vi "Integration_Test_All_Methods.vi"() -> ()   [LabVIEW 2016]
uses:
  <vilib>/httpClient/LabVIEWHTTPClient.lvlib
  Response/Response.lvclass
panel:
  out "GET":string
  out "GET":dbl
  out "Put":bool
  out "PUT":string="{\n  \"id\": 5,\n  \"name\": \"FIveHUNDRED\",\n  \"age\": \"SIXTYTWO\"\n}"
  out "Patch":bool
  out "Post":bool
  out "Delete":bool
  out "GET":bool
  out "PATCH":string="{\n  \"id\": 5,\n  \"name\": \"Five\",\n  \"age\": \"six\"\n}"
  out "Delete":string="{}"
  out "POST":string="{\n  \"id\": 5,\n  \"name\": \"Five\"\n}"
  out "Get":string="[\n  {\n    \"id\": 0,\n    \"name\": \"Zero\",\n    \"age\": \"Zero\"\n  },\n  {\n    \"id\": 1,\n    \"name\": \"one\",\n    \"age\": \"one\"\n  },\n  {\n    \"id\": 2,\n    \"name\": \"two\",\n    \"age\": \"two\"\n  },\n  {\n    \"id\": 3,\n    \"name\": \"three\",\n    \"age\": \"three\"\n  },\n  {\n    \"id\": 4,\n    \"name\": \"four\",\n    \"age\": \"four\"\n  },\n  {\n    \"id\": 5,\n    \"name\": \"five\"\n  }\n]"
  out "LabVIEW Get":string="[\n  {\n    \"id\": 0,\n    \"name\": \"Zero\",\n    \"age\": \"Zero\"\n  },\n  {\n    \"id\": 1,\n    \"name\": \"one\",\n    \"age\": \"one\"\n  },\n  {\n    \"id\": 2,\n    \"name\": \"two\",\n    \"age\": \"two\"\n  },\n  {\n    \"id\": 3,\n    \"name\": \"three\",\n    \"age\": \"three\"\n  },\n  {\n    \"id\": 4,\n    \"name\": \"four\",\n    \"age\": \"four\"\n  },\n  {\n    \"id\": 5,\n    \"name\": \"FIveHUNDRED\",\n    \"age\": \"SIXTYTWO\"\n  }\n]"
  in  "Path to db.json file":path=path "C:/Users/monke/Desktop/db.json"
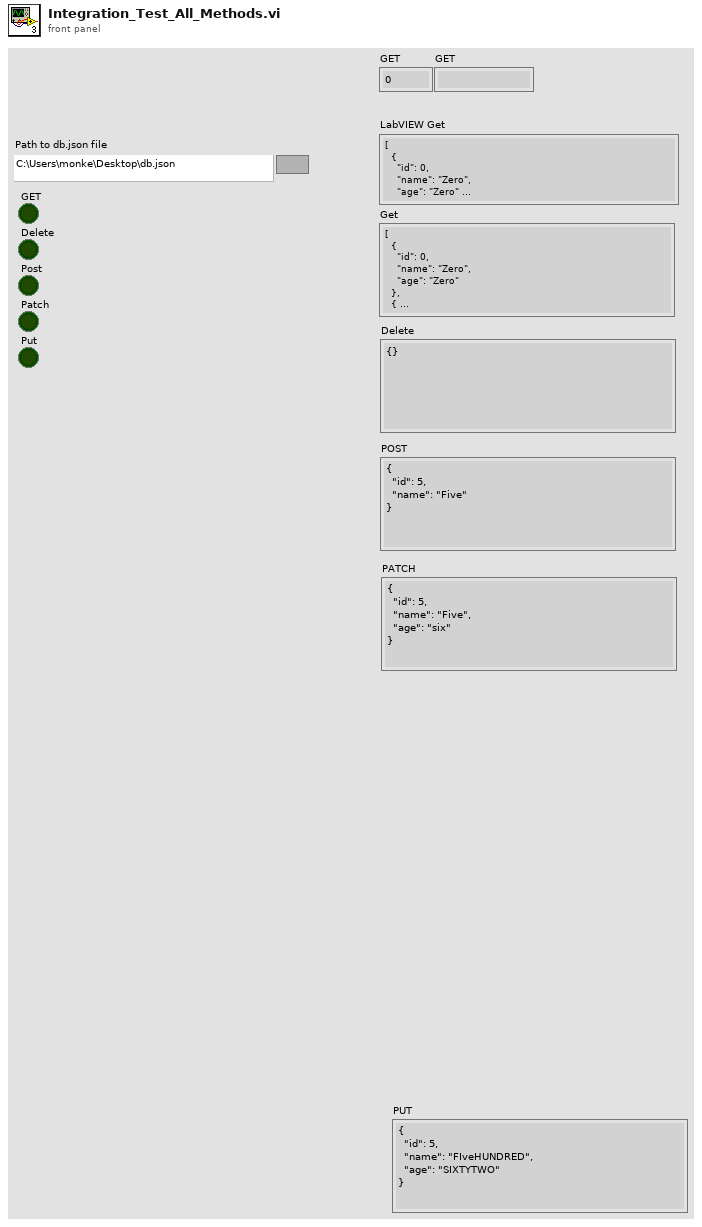
[diagram p1: front panel]
types:
  T1 = enum32{"invalid app kind", "Development System", "Run Time System", "Student Edition", "Embedded LabVIEW", "Evaluation", "Custom"}
  T2 = enum32{"Invalid", "Standard", "Closed", "Hidden", "Minimized", "Maximized"}
  T3 = enum16{"open", "replace", "create", "open or create", "replace or create", "replace or create with confirmation"}
  T4 = cluster{"Core":cluster{"Current VI Reference":refnum<vi>, "Close Panel on Exit?":bool}, "Your Boolean data":bool, "Log":string}
  T5 = cluster{"Current VI Reference":refnum<vi>, "Close Panel on Exit?":bool}
  T6 = typedef "LabVIEWHTTPClient.lvlib/ClientHandle.ctl" = refnum<k1>
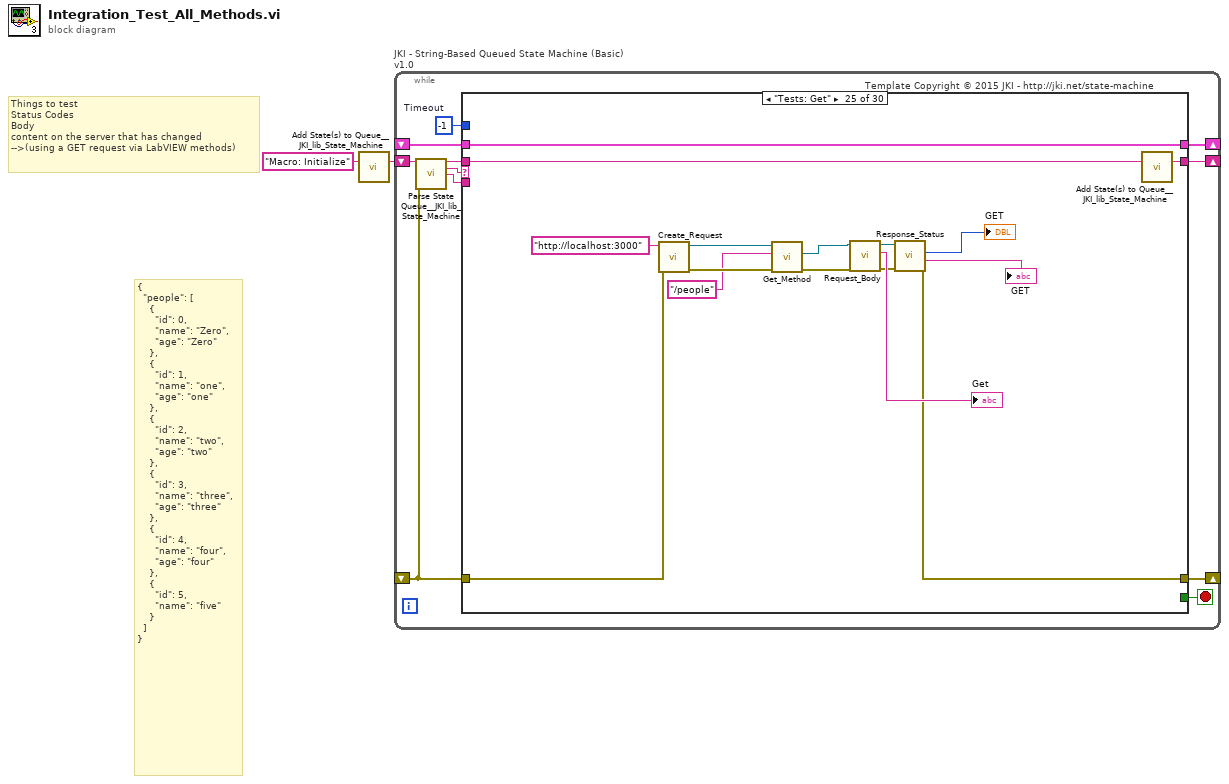
[diagram p0: block diagram]
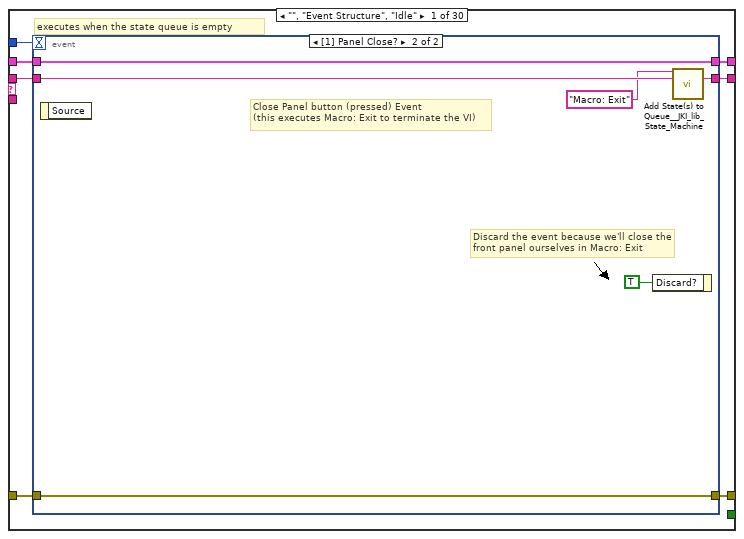
[diagram p2: hidden frame]
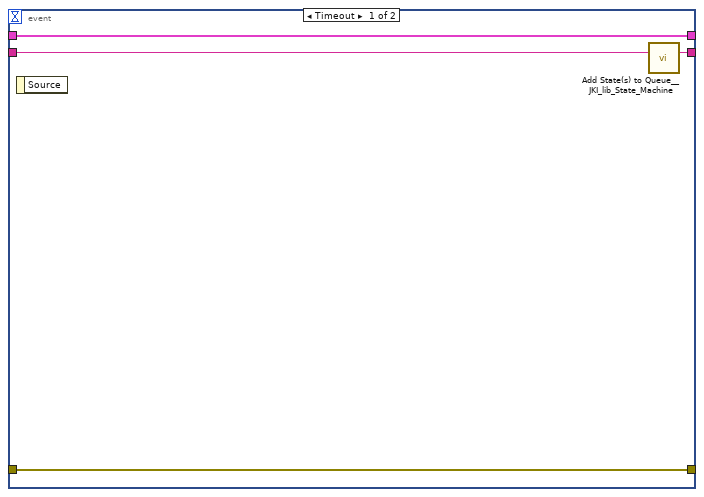
[diagram p3: hidden frame]
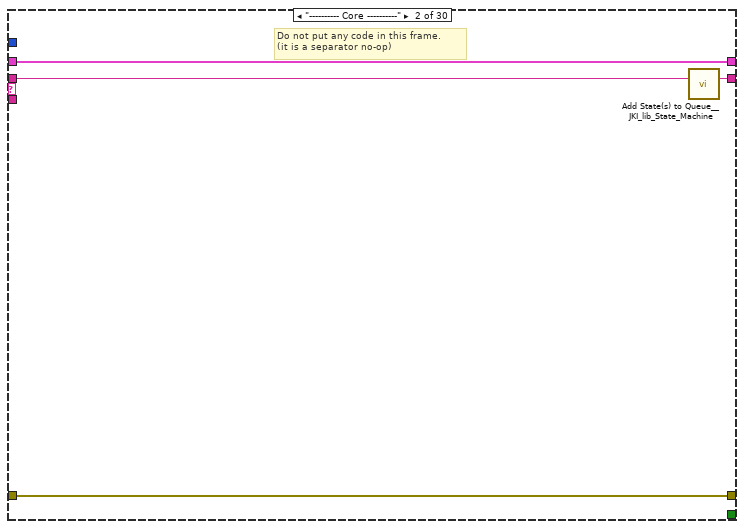
[diagram p4: hidden frame]
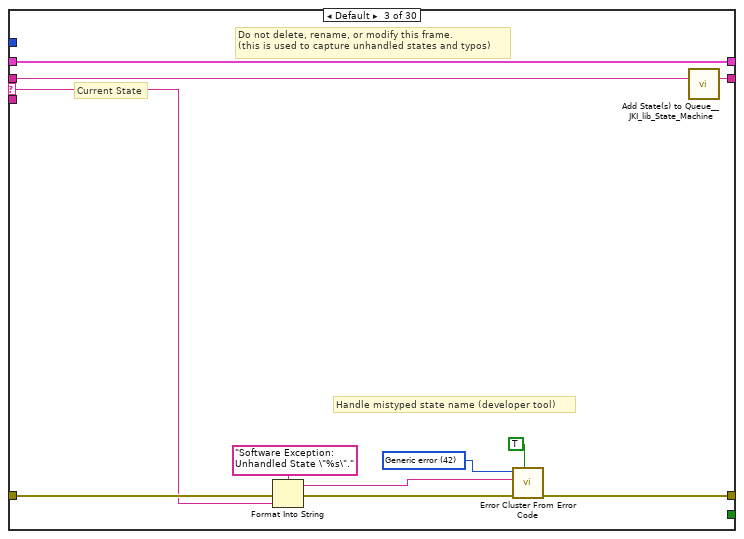
[diagram p5: hidden frame]
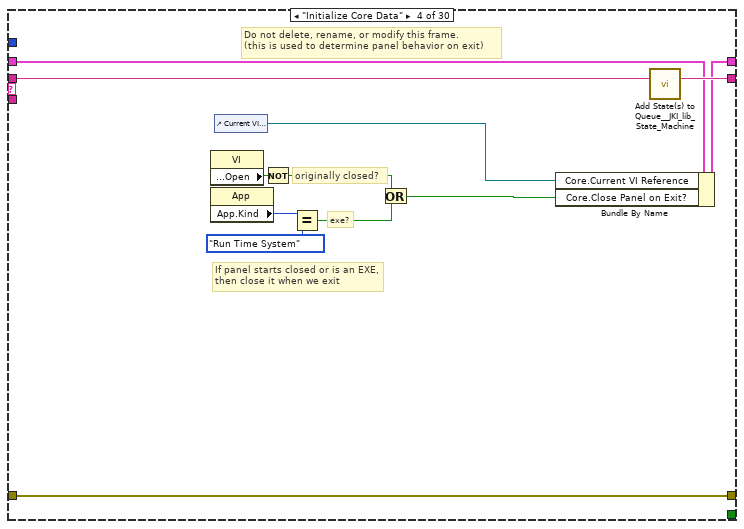
[diagram p6: hidden frame]
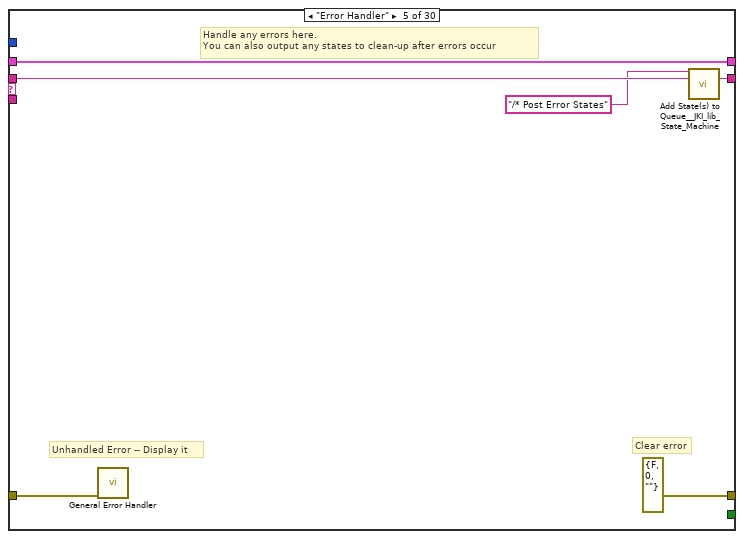
[diagram p7: hidden frame]
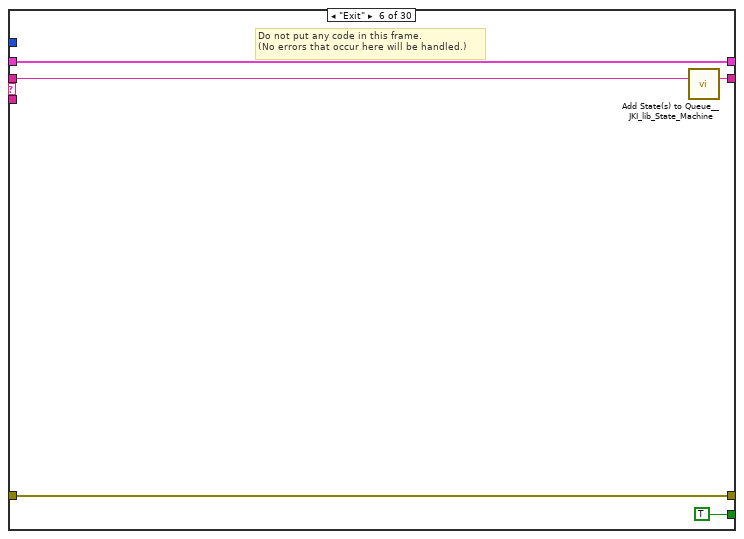
[diagram p8: hidden frame]
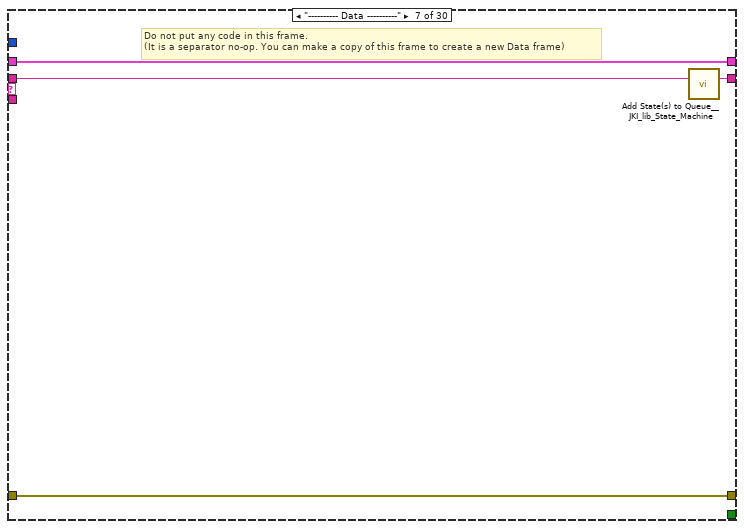
[diagram p9: hidden frame]
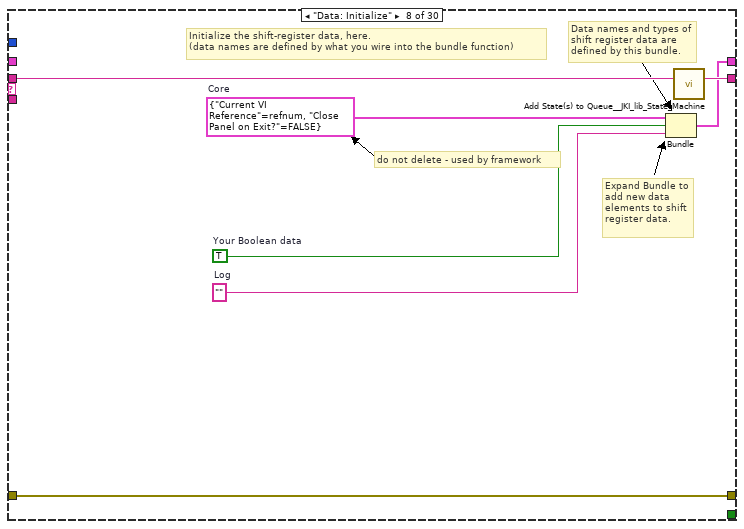
[diagram p10: hidden frame]
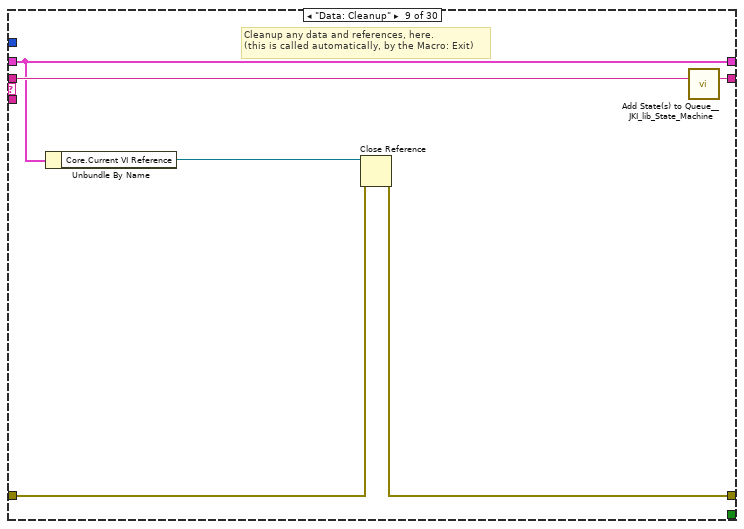
[diagram p11: hidden frame]
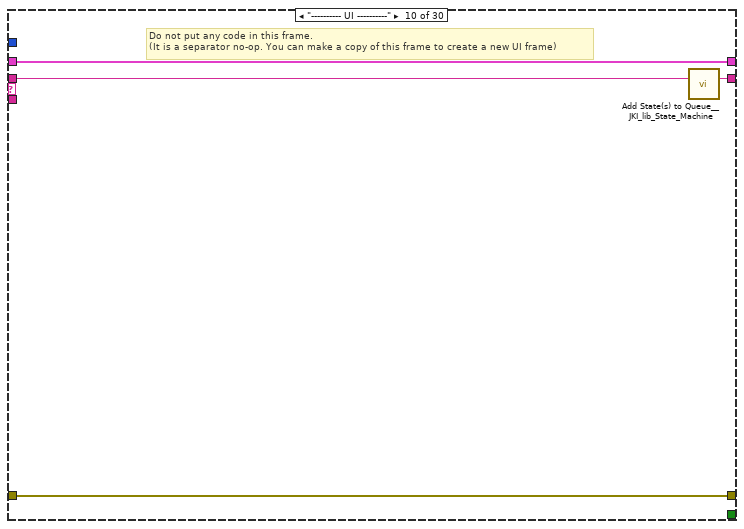
[diagram p12: hidden frame]
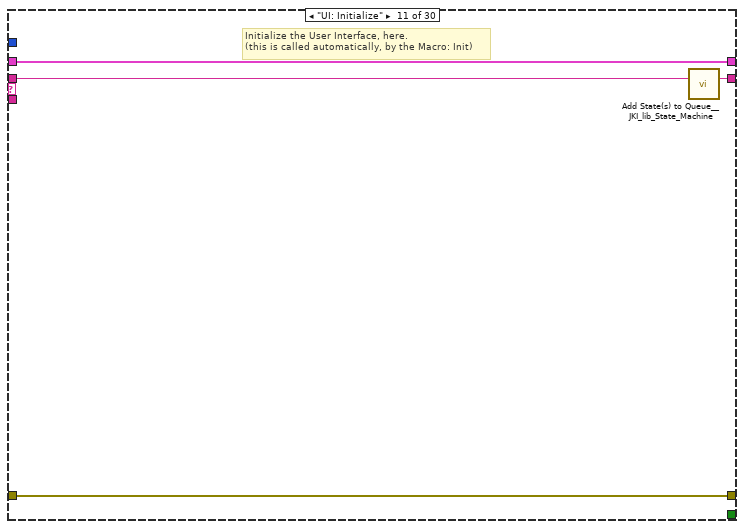
[diagram p13: hidden frame]
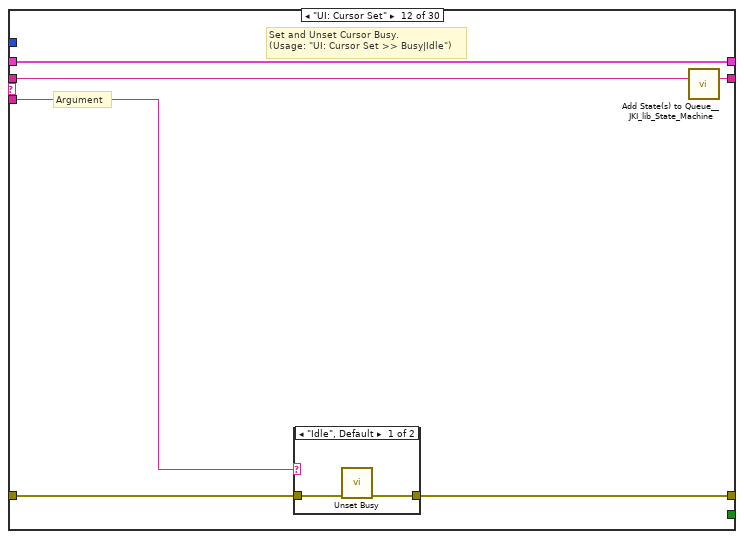
[diagram p14: hidden frame]
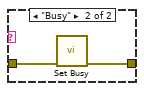
[diagram p15: hidden frame]
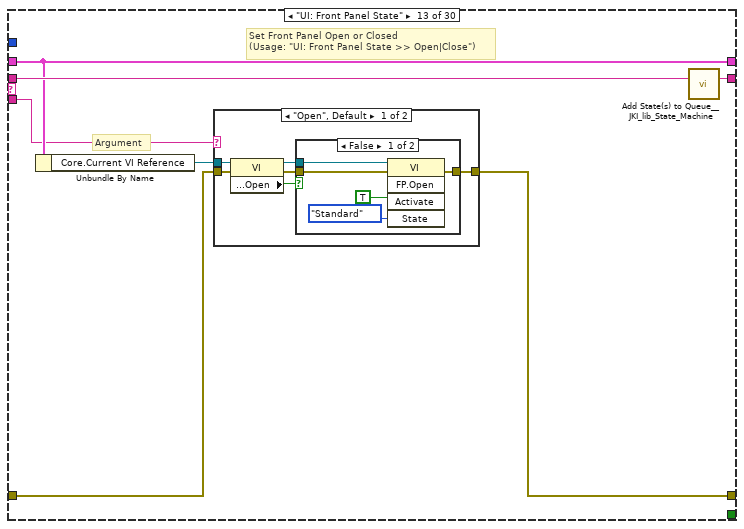
[diagram p16: hidden frame]
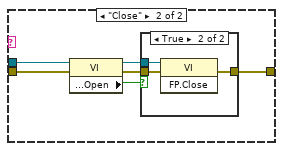
[diagram p18: hidden frame]
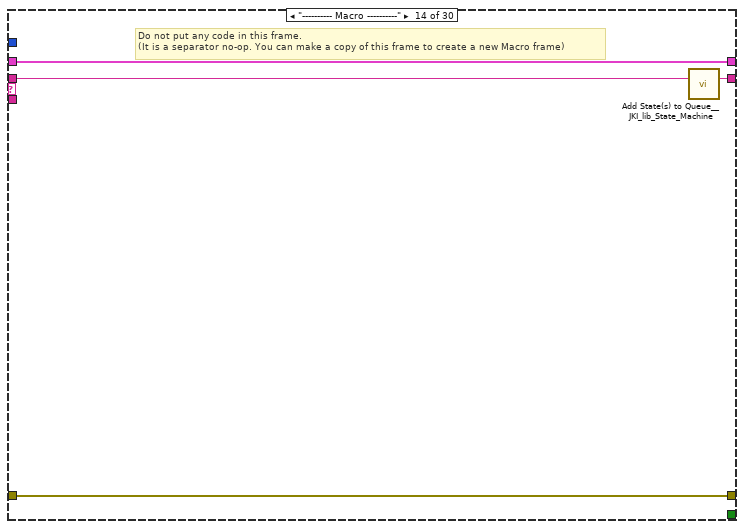
[diagram p20: hidden frame]
diagram:
  # "{\n  \"people\": [\n    {\n      \"id\": 0,\n      \"name\": \"Zero\",\n      \"age\": \"Zero\"\n    },\n    {\n      \"id\": 1,\n      \"name\": \"one\",\n      \"age\": \"one\"\n    },\n    {\n      \"id\": 2,\n      \"name\": \"two\",\n      \"age\": \"two\"\n    },\n    {\n      \"id\": 3,\n      \"name\": \"three\",\n      \"age\": \"three\"\n    },\n    {\n      \"id\": 4,\n      \"name\": \"four\",\n      \"age\": \"four\"\n    },\n    {\n      \"id\": 5,\n      \"name\": \"five\"\n    }\n  ]\n}"
  # "Things to test\nStatus Codes\nBody\ncontent on the server that has changed\n-->(using a GET request via LabVIEW methods)"
  n1 = call <vilib>:"Add State(s) to Queue__JKI_lib_State_Machine.vi"("State(s) in (\"\")"="Macro: Initialize") -> ("States Out"=w2:string)  [unwired: 14 in]
  n2 = while "JKI - String-Based Queued State Machine (Basic) v1.0" {
    shift-right: [w6] -> _
    shift-left: _ -> [w5]
    shift-right: [w9] -> _
    shift-left: _ -> [w3]
    shift-right: [w8] -> _
    shift-left: w2 -> [w10]
    stop <- w7 stop-if-true
    w4 = -1  # Timeout
    # "Template Copyright © 2015 JKI - http://jki.net/state-machine"
    n3 = call <vilib>:"Parse State Queue__JKI_lib_State_Machine.vi"("State Queue"=w10, "Error In (no error)"=w3) -> ("Remaining States"=w12:string, "Current State"=w13:string, "Arguments"=w11:string)  [unwired: 11 in]
    n4 = case shown="\"Tests: Get\"" w13 {
      selector: w13 -> [_ _ w35 _ _ _ _ _ _ _ _ _ _ _ _ _ _ _ _ _ _ _ _ _ _ _ _ _ _ _]
      tunnel: w12 -> [w20 w34 w39 w57 w63 w68 w72 w79 w85 w89 w93 w99 w110 w136 w141 w146 w156 w160 w172 w183 w187 w191 w203 w222 w238 w250 w264 w278 w292 w296]
      tunnel: w11 -> [_ _ _ _ _ _ _ _ _ _ _ w94 w104 _ _ _ _ _ _ _ _ _ w194 _ _ _ _ _ _ _]
      tunnel: w5 -> [w18 w31 w37 w48 w60 w66 w69 _ w80 w86 w91 w97 w106 w133 w138 w143 w153 w158 w170 w181 w184 w188 w192 w219 w225 w248 w262 w276 w290 w293]
      tunnel: [w17 w32 w41 w54 errorcluster {"status"=FALSE, "code"=0, "source"=""} ("error out") w65 w70 w76 w81 w87 w90 w95 w107 w134 w139 w144 w154 w157 w161 w173 w185 w189 w196 w220 w226 w239 w253 w265 w279 w294] -> w9
      tunnel: w3 -> [w16 w32 w40 w54 w59 w65 w70 w76 w82 w87 w90 w96 w108 w134 w139 w144 w154 w157 w162 w174 w185 w189 w197 w220 w233 w240 w254 w266 w280 w294]
      tunnel: [w19 w33 w38 w56 w62 w67 w71 w78 w84 w88 w92 w98 w109 w135 w140 w145 w155 w159 w171 w182 w186 w190 w202 w221 w237 w249 w263 w277 w291 w295] -> w8
      tunnel: [_ _ _ _ _ TRUE _ _ _ _ _ _ _ _ _ _ _ _ _ _ _ _ _ _ _ _ _ _ _ _] -> w7
      tunnel: [w15 w31 w37 w55 w60 w66 w69 w77 w80 w86 w91 w97 w106 w133 w138 w143 w153 w158 w170 w181 w184 w188 w192 w219 w225 w248 w262 w276 w290 w293] -> w6
      tunnel: w4 -> [w14 _ _ _ _ _ _ _ _ _ _ _ _ _ _ _ _ _ _ _ _ _ _ _ _ _ _ _ _ _]
      frame "", "Event Structure", "Idle" {
        # "executes when the state queue is empty"
        n5 = event shown="[1] Panel Close?" {
          selector: _ -> [_ _]
          dyn-events: _ -> [_ _]
          timeout: w14 -> [_ _]
          tunnel: w20 -> [w24 w30]
          tunnel: [w23 w29] -> w19
          tunnel: w18 -> [w21 w27]
          tunnel: [w22 w28] -> w17
          tunnel: w16 -> [w22 w28]
          tunnel: [w21 w27] -> w15
          event Timeout {
            n6 = event-data() -> ()  [unwired: 1 in, 1 out]
            n7 = call <vilib>:"Add State(s) to Queue__JKI_lib_State_Machine.vi"("State(s) in (\"\")"=w24) -> ("States Out"=w23:string)  [unwired: 14 in]
          }
          event Panel Close? {
            # "Discard the event because we'll close the front panel ourselves in Macro: Exit"
            # "Close Panel button (pressed) Event\n(this executes Macro: Exit to terminate the VI)"
            n8 = event-data() -> ()  [unwired: 1 in, 1 out]
            n9 = event-data("Discard?"=TRUE) -> ()  [unwired: 1 in, 1 out]
            n10 = call <vilib>:"Add State(s) to Queue__JKI_lib_State_Machine.vi"("State(s) in Front (\"\")"="Macro: Exit", "State(s) in (\"\")"=w30) -> ("States Out"=w29:string)  [unwired: 13 in]
          }
        }
      }
      frame "---------- Core ----------" {
        # "Do not put any code in this frame.\n(it is a separator no-op)"
        n11 = call <vilib>:"Add State(s) to Queue__JKI_lib_State_Machine.vi"("State(s) in (\"\")"=w34) -> ("States Out"=w33:string)  [unwired: 14 in]
      }
      frame Default {
        w44 = 42 items=["No error", "Argument error", "Memory is full", "Out of zone", "End of file", "File already open", "Generic file I/O error", "File not found", "File permission error", "Disk is full", "Duplicate path", "Too many files open", "System feature not enabled", "Resource file not found", "Cannot add resource", "Resource not found", "Image not found", "Image memory error", "Pen does not exist", "Config type invalid", "Config token not found", "Config parse error", "Config memory error", "Bad external code format", "Bad external code offset", "External code not present", "Null window", "Destroy window error", "Null menu", "Print aborted", "Bad print record", "Print driver error", "Windows error during printing", "Memory error during printing", "Print dialog error", "Generic print error", "Invalid device refnum", "Device not found", "Device parameter error", "Device unit error", "Cannot open device", "Device call aborted", "Generic error", "Cancelled by user", "Object ID too low", "Object ID too high", "Object not in heap", "Unknown heap", "Unknown object (invalid DefProc)", "Unknown object (DefProc not in table)", "Message out of range", "Invalid (null) method", "Unknown message", "Manager call not supported", "Bad address", "Network operation in progress", "Network operation timed out", "Connection is busy", "Network attribute not supported", "Network error", "Address in use", "System out of memory", "Connection aborted", "Connection refused", "Not connected", "Already connected", "Connection closed", "Initialization error (interapplication manager)", "Bad occurrence", "Wait on unbound occurrence handler", "Occurrence queue overflow", "Datalog type conflict", "Unused", "Unrecognized type (interapplication manager)", "Memory corrupt", "Failed to make temporary DLL", "Old CIN version", "Drag socket not found", "Failed to load drop-object", "Failed to register OLE object", "Failed to release OLE object", "Format specifier type mismatch", "Unknown format specifier", "Too few format specifiers", "Too many format specifiers", "Scan failed", "Newer CIN version", "Error converting to variant", "Runtime menu error", "Password tampered", "Variant attribute not found", "Incompatible variant data type", "Event data is not available", "Event Store is not present", "Occurrence is not found", "Event Queue is not created", "Event info is not available", "Refnum passed is NULL", "Error retrieving Class GUID", "Error retrieving CoClass GUID", "Error retrieving TypeLib GUID.", "Bad built application magic bytes.", "Specific driver is different from the specific driver associated with the Logical Name.", "There is no session opened to the class driver.", "Max Error", "MAX - Error with config objects", "MAX - Error loading configuration", "MAX - Group not supported"]
        # "Current State"
        # "Do not delete, rename, or modify this frame.\n(this is used to capture unhandled states and typos)"
        # "Handle mistyped state name (developer tool)"
        n12 = Format Into String(format string="Software Exception: Unhandled State \"%s\"." ("message"), error in=w40, w35) -> (resulting string=w43:string, error out=w42:errorcluster)  [unwired: 1 in]
        n13 = call <vilib>:"Error Cluster From Error Code.vi"("show call chain? (False)"=TRUE, "error in (no error)"=w42, "error message (\"\")"=w43, "error code (0)"=w44) -> ("error out"=w41:errorcluster)  [unwired: 5 in]
        n14 = call <vilib>:"Add State(s) to Queue__JKI_lib_State_Machine.vi"("State(s) in (\"\")"=w39) -> ("States Out"=w38:string)  [unwired: 14 in]
      }
      frame "Initialize Core Data" {
        # "Do not delete, rename, or modify this frame.\n(this is used to determine panel behavior on exit)"
        # "originally closed?"
        # "exe?"
        # "If panel starts closed or is an EXE, then close it when we exit"
        n15 = property class="VI"() -> ("Front Panel.Open"=w53:bool)  [unwired: 2 in, 2 out]
        n16 = property class="App"() -> ("App.Kind"=w52:T1)  [unwired: 2 in, 2 out]
        n17 = control-ref of="Current VI Reference"() -> (w46:refnum<vi>)
        n18 = Not(x=w53) -> (.not. x?=w50:bool)
        n19 = Equal?(x=w52, y=T1."Run Time System" ("Application:Kind")) -> (x = y?=w49:bool)
        n20 = Or(x=w50, y=w49) -> (x .or. y?=w47:bool)
        n21 = Bundle By Name(cluster=w48, "Core.Current VI Reference"=w46, "Core.Close Panel on Exit?"=w47) -> (w55:T4)
        n22 = call <vilib>:"Add State(s) to Queue__JKI_lib_State_Machine.vi"("State(s) in (\"\")"=w57) -> ("States Out"=w56:string)  [unwired: 14 in]
      }
      frame "Error Handler" {
        # "Unhandled Error -- Display it"
        # "Handle any errors here.\nYou can also output any states to clean-up after errors occur"
        # "Clear error"
        n23 = call <vilib>:"General Error Handler.vi"("error in (no error)"=w59) -> ()  [unwired: 10 in, 5 out]
        n24 = call <vilib>:"Add State(s) to Queue__JKI_lib_State_Machine.vi"("State(s) in Front (\"\")"="/* Post Error States", "State(s) in (\"\")"=w63) -> ("States Out"=w62:string)  [unwired: 13 in]
      }
      frame "Exit" {
        # "Do not put any code in this frame.\n(No errors that occur here will be handled.)"
        n25 = call <vilib>:"Add State(s) to Queue__JKI_lib_State_Machine.vi"("State(s) in (\"\")"=w68) -> ("States Out"=w67:string)  [unwired: 14 in]
      }
      frame "---------- Data ----------" {
        # "Do not put any code in this frame.\n(It is a separator no-op. You can make a copy of this frame to create a new Data frame)"
        n26 = call <vilib>:"Add State(s) to Queue__JKI_lib_State_Machine.vi"("State(s) in (\"\")"=w72) -> ("States Out"=w71:string)  [unwired: 14 in]
      }
      frame "Data: Initialize" {
        w73 = T5 {"Current VI Reference"=refnum, "Close Panel on Exit?"=FALSE}  # Core
        w75 = TRUE  # Your Boolean data
        w74 = ""  # Log
        # "do not delete - used by framework"
        # "Expand Bundle to add new data elements to shift register data."
        # "Data names and types of shift register data are defined by this bundle."
        # "Initialize the shift-register data, here.\n(data names are defined by what you wire into the bundle function)"
        n27 = Bundle("Core"=w73, "Your Boolean data"=w75, "Log"=w74) -> (w77:T4)  [unwired: 1 in]
        n28 = call <vilib>:"Add State(s) to Queue__JKI_lib_State_Machine.vi"("State(s) in (\"\")"=w79) -> ("States Out"=w78:string)  [unwired: 14 in]
      }
      frame "Data: Cleanup" {
        # "Cleanup any data and references, here.\n(this is called automatically, by the Macro: Exit)"
        n29 = Unbundle By Name(w80) -> ("Core.Current VI Reference"=w83:refnum<vi>)
        n30 = Close Reference(reference=w83, error in (no error)=w82) -> (error out=w81:errorcluster)
        n31 = call <vilib>:"Add State(s) to Queue__JKI_lib_State_Machine.vi"("State(s) in (\"\")"=w85) -> ("States Out"=w84:string)  [unwired: 14 in]
      }
      frame "---------- UI ----------" {
        # "Do not put any code in this frame.\n(It is a separator no-op. You can make a copy of this frame to create a new UI frame)"
        n32 = call <vilib>:"Add State(s) to Queue__JKI_lib_State_Machine.vi"("State(s) in (\"\")"=w89) -> ("States Out"=w88:string)  [unwired: 14 in]
      }
      frame "UI: Initialize" {
        # "Initialize the User Interface, here.\n(this is called automatically, by the Macro: Init)"
        n33 = call <vilib>:"Add State(s) to Queue__JKI_lib_State_Machine.vi"("State(s) in (\"\")"=w93) -> ("States Out"=w92:string)  [unwired: 14 in]
      }
      frame "UI: Cursor Set" {
        # "Argument"
        # "Set and Unset Cursor Busy.\n(Usage: \"UI: Cursor Set >> Busy|Idle\")"
        n34 = case shown="\"Idle\", Default" w94 {
          tunnel: w96 -> [w101 w103]
          tunnel: [w100 w102] -> w95
          frame "Idle", Default {
            n35 = call <vilib>:"Unset Busy.vi"("error in (no error)"=w101) -> ("error out"=w100:errorcluster)  [unwired: 10 in]
          }
          frame "Busy" {
            n36 = call <vilib>:"Set Busy.vi"("error in (no error)"=w103) -> ("error out"=w102:errorcluster)  [unwired: 9 in, 1 out]
          }
        }
        n37 = call <vilib>:"Add State(s) to Queue__JKI_lib_State_Machine.vi"("State(s) in (\"\")"=w99) -> ("States Out"=w98:string)  [unwired: 14 in]
      }
      frame "UI: Front Panel State" {
        # "Argument"
        # "Set Front Panel Open or Closed\n(Usage: \"UI: Front Panel State >> Open|Close\")"
        n38 = Unbundle By Name(w106) -> ("Core.Current VI Reference"=w105:refnum<vi>)
        n39 = case shown="\"Open\", Default" w104 {
          tunnel: w108 -> [w114 w127]
          tunnel: [w116 w128] -> w107
          tunnel: w105 -> [w115 w125]
          frame "Open", Default {
            n40 = property class="VI"(reference=w115, error in=w114) -> (reference out=w112:refnum<vi>, error out=w113:errorcluster, "Front Panel.Open"=w111:bool)
            n41 = case shown="False" w111 {
              tunnel: [w119 w122] -> w116
              tunnel: w113 -> [w118 w122]
              tunnel: w112 -> [w117 _]
              frame False {
                n42 = invoke class="VI" method="FP.Open"(reference=w117, error in=w118, "Activate"=TRUE, "State"=T2."Standard") -> (error out=w119:errorcluster)  [unwired: 1 in, 4 out]
              }
              frame True {
              }
            }
          }
          frame "Close" {
            n43 = property class="VI"(reference=w125, error in=w127) -> (reference out=w124:refnum<vi>, error out=w126:errorcluster, "Front Panel.Open"=w123:bool)
            n44 = case shown="True" w123 {
              tunnel: [w129 w132] -> w128
              tunnel: w126 -> [w129 w131]
              tunnel: w124 -> [_ w130]
              frame False {
              }
              frame True {
                n45 = invoke class="VI" method="FP.Close"(reference=w130, error in=w131) -> (error out=w132:errorcluster)  [unwired: 1 in, 2 out]
              }
            }
          }
        }
        n46 = call <vilib>:"Add State(s) to Queue__JKI_lib_State_Machine.vi"("State(s) in (\"\")"=w110) -> ("States Out"=w109:string)  [unwired: 14 in]
      }
      frame "---------- Macro ----------" {
        # "Do not put any code in this frame.\n(It is a separator no-op. You can make a copy of this frame to create a new Macro frame)"
        n47 = call <vilib>:"Add State(s) to Queue__JKI_lib_State_Machine.vi"("State(s) in (\"\")"=w136) -> ("States Out"=w135:string)  [unwired: 14 in]
      }
      frame "Macro: Initialize" {
        w137 = "Data: Initialize\nInitialize Core Data\nUI: Initialize\nJsonServer: Create_File\nJsonServer: Run\nUI: Front Panel State >> Open\nMacro: Run Tests"  # Data: Initialize Initialize Core Data UI: Initialize JsonServer: Create_File JsonServer: Run UI: Front Panel State >> Open Macro: Run Tests
        # "Initialization Macro\n(This is called once, when the VI starts)"
        n48 = call <vilib>:"Add State(s) to Queue__JKI_lib_State_Machine.vi"("State(s) in Front (\"\")"=w137, "State(s) in (\"\")"=w141) -> ("States Out"=w140:string)  [unwired: 13 in]
      }
      frame "Macro: Run Tests" {
        # "Do not put any code in this frame.\n(It is a separator no-op. You can make a copy of this frame to create a new Macro frame)"
        n49 = call <vilib>:"Add State(s) to Queue__JKI_lib_State_Machine.vi"("State(s) in Front (\"\")"="Tests: Get\nLabVIEW: Get>>get\nTests: Delete\nLabVIEW: Get>>delete\nTests: Post\nLabVIEW: Get>>post\nTests: Patch\nLabVIEW: Get>>patch\nTests: Put\nLabVIEW: Get>>put\n//Tests: Head", "State(s) in (\"\")"=w146) -> ("States Out"=w145:string)  [unwired: 13 in]
      }
      frame "Macro: Exit" {
        # "Exit Macro\n(This is called once, when the VI exits)"
        n50 = Unbundle By Name(w153) -> ("Core.Close Panel on Exit?"=w152:bool)
        n51 = Select(t="UI: Front Panel State >> Close", s=w152, f="") -> (s? t:f=w149:string)
        n52 = call <vilib>:"Add State(s) to Queue__JKI_lib_State_Machine.vi"("State(s) in (\"\")"=w149, "State(s) at Back (\"\")"="Data: Cleanup\nExit") -> ("States Out"=w147:string)  [unwired: 13 in]
        n53 = call <vilib>:"Add State(s) to Queue__JKI_lib_State_Machine.vi"("State(s) in Front (\"\")"=w147, "State(s) in (\"\")"=w156) -> ("States Out"=w155:string)  [unwired: 13 in]
      }
      frame "---------- JsonServer ----------" {
        n54 = call <vilib>:"Add State(s) to Queue__JKI_lib_State_Machine.vi"("State(s) in (\"\")"=w160) -> ("States Out"=w159:string)  [unwired: 14 in]
      }
      frame "JsonServer: Create_File" {
        n55 = Open/Create/Replace File(file path (use dialog)=path "C:/Users/monke/Desktop/db.json", error in=w162, operation (0:open)=T3."replace or create") -> (refnum out=w166:refnum<file>, error out=w163:errorcluster)  [unwired: 3 in, 1 out]
        n56 = Write to Text File(file (use dialog)=w166, text="{\n  \"people\": [\n    {\n      \"id\": 0,\n      \"name\": \"Zero\",\n      \"age\": \"Zero\"\n    },\n    {\n      \"id\": 1,\n      \"name\": \"one\",\n      \"age\": \"one\"\n    },\n    {\n      \"id\": 2,\n      \"name\": \"two\",\n      \"age\": \"two\"\n    },\n    {\n      \"id\": 3,\n      \"name\": \"three\",\n      \"age\": \"three\"\n    },\n    {\n      \"id\": 4,\n      \"name\": \"four\",\n      \"age\": \"four\"\n    },\n    {\n      \"id\": 5,\n      \"name\": \"five\"\n    }\n  ]\n}", error in=w163) -> (refnum out=w165:refnum<file>, error out=w164:errorcluster)  [unwired: 1 in, 1 out]
        n57 = Close File(refnum=w165, error in=w164) -> (error out=w161:errorcluster)  [unwired: 1 out]
        n58 = call <vilib>:"Add State(s) to Queue__JKI_lib_State_Machine.vi"("State(s) in (\"\")"=w172) -> ("States Out"=w171:string)  [unwired: 14 in]
      }
      frame "JsonServer: Run" {
        # "Make sure to add db.json file to local directory then change this state."
        n59 = Strip Path(path="Path to db.json file") -> (stripped path=w179:path)  [unwired: 1 out]
        n60 = call <vilib>:"System Exec.vi"("wait until completion? (T)"=FALSE, "error in (no error)"=w174, "working directory"=w179, "command line"="cmd /c json-server db.json") -> ("error out"=w176:errorcluster)  [unwired: 4 in, 3 out]
        n61 = call <userlib>:"Wait (ms)__ogtk.vi"("error in (no error)"=w176, "milliseconds to wait"=u32 10000) -> ("error out"=w173:errorcluster)  [unwired: 8 in, 1 out]
        n62 = call <vilib>:"Add State(s) to Queue__JKI_lib_State_Machine.vi"("State(s) in (\"\")"=w183) -> ("States Out"=w182:string)  [unwired: 14 in]
      }
      frame "---------- LabVIEW ----------" {
        n63 = call <vilib>:"Add State(s) to Queue__JKI_lib_State_Machine.vi"("State(s) in (\"\")"=w187) -> ("States Out"=w186:string)  [unwired: 14 in]
      }
      frame "LabVIEW: Head" {
        n64 = call <vilib>:"Add State(s) to Queue__JKI_lib_State_Machine.vi"("State(s) in (\"\")"=w191) -> ("States Out"=w190:string)  [unwired: 14 in]
      }
      frame "LabVIEW: Get" {
        n65 = call <vilib>:"OpenHandle.vi"("error in (no error)"=w197) -> ("client handle out"=w201:T6, "error out"=w198:errorcluster)  [unwired: 13 in]
        n66 = call <vilib>:"GET.vi"("client handle"=w201, "url"="http://localhost:3000/people", "error in (no error)"=w198) -> ("client handle out"=w200:T6, "body"=w193:string, "error out"=w199:errorcluster)  [unwired: 9 in, 1 out]
        "LabVIEW Get" <- w193
        n67 = call <vilib>:"CloseHandle.vi"("client handle"=w200, "error in (no error)"=w199) -> ("error out"=w196:errorcluster)  [unwired: 13 in]
        n68 = case shown="\"get\", Default" w194 {
          tunnel: w193 -> [w204 w208 w211 w214 w217]
          frame "get", Default {
            n69 = Equal?(x=w204, y="[\n  {\n    \"id\": 0,\n    \"name\": \"Zero\",\n    \"age\": \"Zero\"\n  },\n  {\n    \"id\": 1,\n    \"name\": \"one\",\n    \"age\": \"one\"\n  },\n  {\n    \"id\": 2,\n    \"name\": \"two\",\n    \"age\": \"two\"\n  },\n  {\n    \"id\": 3,\n    \"name\": \"three\",\n    \"age\": \"three\"\n  },\n  {\n    \"id\": 4,\n    \"name\": \"four\",\n    \"age\": \"four\"\n  },\n  {\n    \"id\": 5,\n    \"name\": \"five\"\n  }\n]") -> (x = y?=→"GET":bool)
          }
          frame "delete" {
            n70 = Equal?(x=w208, y="[\n  {\n    \"id\": 0,\n    \"name\": \"Zero\",\n    \"age\": \"Zero\"\n  },\n  {\n    \"id\": 1,\n    \"name\": \"one\",\n    \"age\": \"one\"\n  },\n  {\n    \"id\": 2,\n    \"name\": \"two\",\n    \"age\": \"two\"\n  },\n  {\n    \"id\": 3,\n    \"name\": \"three\",\n    \"age\": \"three\"\n  },\n  {\n    \"id\": 4,\n    \"name\": \"four\",\n    \"age\": \"four\"\n  }\n]") -> (x = y?=→"Delete":bool)
          }
          frame "post" {
            n71 = Equal?(x=w211, y="[\n  {\n    \"id\": 0,\n    \"name\": \"Zero\",\n    \"age\": \"Zero\"\n  },\n  {\n    \"id\": 1,\n    \"name\": \"one\",\n    \"age\": \"one\"\n  },\n  {\n    \"id\": 2,\n    \"name\": \"two\",\n    \"age\": \"two\"\n  },\n  {\n    \"id\": 3,\n    \"name\": \"three\",\n    \"age\": \"three\"\n  },\n  {\n    \"id\": 4,\n    \"name\": \"four\",\n    \"age\": \"four\"\n  },\n  {\n    \"id\": 5,\n    \"name\": \"Five\"\n  }\n]") -> (x = y?=→"Post":bool)
          }
          frame "patch" {
            n72 = Equal?(x=w214, y="[\n  {\n    \"id\": 0,\n    \"name\": \"Zero\",\n    \"age\": \"Zero\"\n  },\n  {\n    \"id\": 1,\n    \"name\": \"one\",\n    \"age\": \"one\"\n  },\n  {\n    \"id\": 2,\n    \"name\": \"two\",\n    \"age\": \"two\"\n  },\n  {\n    \"id\": 3,\n    \"name\": \"three\",\n    \"age\": \"three\"\n  },\n  {\n    \"id\": 4,\n    \"name\": \"four\",\n    \"age\": \"four\"\n  },\n  {\n    \"id\": 5,\n    \"name\": \"Five\",\n    \"age\": \"six\"\n  }\n]") -> (x = y?=→"Patch":bool)
          }
          frame "put" {
            n73 = Equal?(x=w217, y="[\n  {\n    \"id\": 0,\n    \"name\": \"Zero\",\n    \"age\": \"Zero\"\n  },\n  {\n    \"id\": 1,\n    \"name\": \"one\",\n    \"age\": \"one\"\n  },\n  {\n    \"id\": 2,\n    \"name\": \"two\",\n    \"age\": \"two\"\n  },\n  {\n    \"id\": 3,\n    \"name\": \"three\",\n    \"age\": \"three\"\n  },\n  {\n    \"id\": 4,\n    \"name\": \"four\",\n    \"age\": \"four\"\n  },\n  {\n    \"id\": 5,\n    \"name\": \"FIveHUNDRED\",\n    \"age\": \"SIXTYTWO\"\n  }\n]") -> (x = y?=→"Put":bool)
          }
        }
        n74 = call <vilib>:"Add State(s) to Queue__JKI_lib_State_Machine.vi"("State(s) in (\"\")"=w203) -> ("States Out"=w202:string)  [unwired: 14 in]
      }
      frame "---------- Tests ----------" {
        n75 = call <vilib>:"Add State(s) to Queue__JKI_lib_State_Machine.vi"("State(s) in (\"\")"=w222) -> ("States Out"=w221:string)  [unwired: 14 in]
      }
      frame "Tests: Get" {
        n76 = call "Create_Request.vi"("error in (no error)"=w233, "Base URL"="http://localhost:3000") -> ("error out"=w234:errorcluster, "Request out"=w235:refnum<class "Request.lvclass">)  [unwired: 8 in]
        n77 = call "Get_Method.vi"("error in (no error)"=w234, "Endpoint URL"="/people", "Request in"=w235) -> ("error out"=w231:errorcluster, "Response out"=w232:refnum<class "Response.lvclass">)  [unwired: 6 in, 1 out]
        n78 = call "Request_Body.vi"("error in (no error)"=w231, "Response in"=w232) -> ("error out"=w227:errorcluster, "Response Body"=→"Get":string, "Response out"=w228:refnum<class "Response.lvclass">)  [unwired: 7 in]
        n79 = call "Response_Status.vi"("error in (no error)"=w227, "Response in"=w228) -> ("error out"=w226:errorcluster, "Status Description"=→"GET":string, "Status Code"=→"GET":i32)  [unwired: 6 in, 1 out]
        n80 = call <vilib>:"Add State(s) to Queue__JKI_lib_State_Machine.vi"("State(s) in (\"\")"=w238) -> ("States Out"=w237:string)  [unwired: 14 in]
      }
      frame "Tests: Delete" {
        # "Delete the fifth person"
        n81 = call "Create_Request.vi"("error in (no error)"=w240, "Base URL"="http://localhost:3000") -> ("error out"=w244:errorcluster, "Request out"=w246:refnum<class "Request.lvclass">)  [unwired: 8 in]
        n82 = call "Delete_Method.vi"("error in (no error)"=w244, "Endpoint URL"="/people/5/", "Request in"=w246) -> ("error out"=w242:errorcluster, "Response out"=w243:refnum<class "Response.lvclass">)  [unwired: 6 in, 1 out]
        n83 = call "Request_Body.vi"("error in (no error)"=w242, "Response in"=w243) -> ("error out"=w239:errorcluster, "Response Body"=→"Delete":string)  [unwired: 7 in, 1 out]
        n84 = call <vilib>:"Add State(s) to Queue__JKI_lib_State_Machine.vi"("State(s) in (\"\")"=w250) -> ("States Out"=w249:string)  [unwired: 14 in]
      }
      frame "Tests: Post" {
        # "Post a new fifth person without age data"
        n85 = call "Create_Request.vi"("error in (no error)"=w254, "Base URL"="http://localhost:3000") -> ("error out"=w258:errorcluster, "Request out"=w260:refnum<class "Request.lvclass">)  [unwired: 8 in]
        n86 = call "Post_Method.vi"("Body Content-Type"="application/json", "error in (no error)"=w258, "Body"=" {\"id\": 5,\"name\": \"Five\"}", "Endpoint URL"="/people", "Request in"=w260) -> ("error out"=w256:errorcluster, "Response out"=w257:refnum<class "Response.lvclass">)  [unwired: 4 in, 1 out]
        n87 = call "Request_Body.vi"("error in (no error)"=w256, "Response in"=w257) -> ("error out"=w253:errorcluster, "Response Body"=→"POST":string)  [unwired: 7 in, 1 out]
        n88 = call <vilib>:"Add State(s) to Queue__JKI_lib_State_Machine.vi"("State(s) in (\"\")"=w264) -> ("States Out"=w263:string)  [unwired: 14 in]
      }
      frame "Tests: Patch" {
        # "body: {\"age\":\"six\"}"
        # "Patch the fifth person to change the age data"
        n89 = call "Create_Request.vi"("error in (no error)"=w266, "Base URL"="http://localhost:3000") -> ("error out"=w272:errorcluster, "Request out"=w274:refnum<class "Request.lvclass">)  [unwired: 8 in]
        n90 = call "Patch_Method.vi"("Body Content-Type"="application/json", "error in (no error)"=w272, "Body"="{\"age\":\"six\"}", "Endpoint URL"="/people/5/", "Request in"=w274) -> ("error out"=w270:errorcluster, "Response out"=w271:refnum<class "Response.lvclass">)  [unwired: 4 in, 1 out]
        n91 = call "Request_Body.vi"("error in (no error)"=w270, "Response in"=w271) -> ("error out"=w265:errorcluster, "Response Body"=→"PATCH":string)  [unwired: 7 in, 1 out]
        n92 = call <vilib>:"Add State(s) to Queue__JKI_lib_State_Machine.vi"("State(s) in (\"\")"=w278) -> ("States Out"=w277:string)  [unwired: 14 in]
      }
      frame "Tests: Put" {
        # "Totally change the entire fifth person with totallydifferent parameters"
        n93 = call "Create_Request.vi"("error in (no error)"=w280, "Base URL"="http://localhost:3000") -> ("error out"=w286:errorcluster, "Request out"=w288:refnum<class "Request.lvclass">)  [unwired: 8 in]
        n94 = call "Put_Method.vi"("Body Content-Type"="application/json", "error in (no error)"=w286, "Body"="{\"id\": 5,\"name\": \"FIveHUNDRED\",\"age\": \"SIXTYTWO\"}", "Endpoint URL"="/people/5/", "Request in"=w288) -> ("error out"=w284:errorcluster, "Response out"=w285:refnum<class "Response.lvclass">)  [unwired: 4 in, 1 out]
        n95 = call "Request_Body.vi"("error in (no error)"=w284, "Response in"=w285) -> ("error out"=w279:errorcluster, "Response Body"=→"PUT":string)  [unwired: 7 in, 1 out]
        n96 = call <vilib>:"Add State(s) to Queue__JKI_lib_State_Machine.vi"("State(s) in (\"\")"=w292) -> ("States Out"=w291:string)  [unwired: 14 in]
      }
      frame "Tests: Head" {
        n97 = call <vilib>:"Add State(s) to Queue__JKI_lib_State_Machine.vi"("State(s) in (\"\")"=w296) -> ("States Out"=w295:string)  [unwired: 14 in]
      }
    }
  }
